vi "Test App Add Process with Used Name Throws Error.vi"(8 "error in (no error)":errorcluster, 11 "Rig Test in":refnum<class "Application Dev Test.lvclass">) -> (0 "error out":errorcluster, 3 "Rig Test out":refnum<class "Application Dev Test.lvclass">)   [LabVIEW 2020, in "Application Dev Test.lvclass"]
uses:
  Application Dev Test.lvclass
  C:/Program Files (x86)/National Instruments/LabVIEW 2020/vi.lib/Astemes/LUnit/Test Case.lvclass
  source/Framework/Process/Process.lvclass
  source/Framework Test Suite/Mock Error Handler/Mock Error Handler.lvclass
  C:/Git/triarc-framework/source/Framework/Error Handler Interface/Error Handler Interface.lvclass
  source/Framework/Process/Process.lvclass/Process.ctl
  source/Framework/Application/Application.lvclass/Application.ctl
  <vilib>/Astemes/LUnit/Test Case.lvclass/Test Case.ctl
  <vilib>/Astemes/LUnit/LUnit Assertion Result.lvclass/LUnit Assertion Result.ctl
  <vilib>/Astemes/LUnit/LUnit Test Case Result.lvclass/LUnit Test Case Result.ctl
  <vilib>/Astemes/LUnit/LUnit Method Result.lvclass/LUnit Method Result.ctl
  b0215dd9-40b6-4c3d-8097-4c1eb93856a7.vi
  source/Framework/Process/Protected/Messaging/Enqueue Message.vi
  source/Framework/Process/Public/Lifecycle/Get Lifecycle State.vi
  source/Framework/Process/Protected/Messaging/Request Message.vi
  source/Framework/Application/Private/Add Process to Map.vi
  source/Framework/Application/Private/Start Idle Processes if Running.vi
  source/Framework/Application/Private/Throw Error If Process Already in App.vi
  source/Framework/Process/Protected/SubVIs/Set Context.vi
  <vilib>/Astemes/LUnit/Palette/Fail.vi
  <vilib>/Astemes/LUnit/Palette/Pass.vi
  <vilib>/Astemes/LUnit/Set Assertion Type.vi
  <vilib>/Astemes/LUnit/Compare Variants.vi
  <vilib>/Astemes/LUnit/Describe Comparison.vi
  source/Framework/Process/Private/SubVIs/Wait for finish.vi
  source/Framework/Process/Private/SubVIs/Set Lifecycle State.vi
  source/Framework/Process/Private/SubVIs/Handle Debug Data.vi
  <vilib>/Utility/error.llb/Clear Errors.vi
  source/Framework/Process/Private/SubVIs/Enqueue Request Message.vi
  source/Framework/Application/Public/Get Process.vi
  source/Framework/Process/Public/Lifecycle/Leave Process Loop.vi
  <vilib>/Astemes/LUnit/Add test result.vi
  <vilib>/Astemes/LUnit/LUnit Write Passed.vi
  <vilib>/Astemes/LUnit/LUnit Write Message.vi
  <vilib>/Astemes/LUnit/LUnit Write Description.vi
  <vilib>/Astemes/LUnit/LUnit Write Assertion Type.vi
  <vilib>/Astemes/LUnit/Variant to string.vi
  source/Framework/Logging/Log Debug.vi
  <vilib>/AdvancedString/1D String Array to Delimited String.vi
  <vilib>/Utility/High Resolution Relative Seconds.vi
  source/Framework/Application/Private/Retrieve Process from App.vi
  source/Framework/Application/Private/Parse Process Name.vi
  source/Framework/Application/Private/Get Process from Map.vi
  <vilib>/Astemes/LUnit/LUnit Record Assertion Result.vi
  <vilib>/AdvancedString/Delimited String to 1D String Array.vi
  <vilib>/Astemes/LUnit/LUnit Aggregate Assertion Results.vi
  <vilib>/Astemes/LUnit/Assertion Result/LUnit Read Status.vi
  <vilib>/Astemes/LUnit/LUnit Read Message.vi
  <vilib>/Astemes/LUnit/LUnit Read Description.vi
  <vilib>/Astemes/LUnit/Method Result/LUnit Merge Status.vi
  <vilib>/Astemes/LUnit/LUnit Concatenate result strings.vi
  source/Framework/Application/Application.lvclass
  C:/Git/triarc-framework/source/Framework/Process/Process.lvclass
  <vilib>/Utility/error.llb/Error Cluster From Error Code.vi
  source/Framework/Process/Public/Read Name.vi
  source/Framework/Process/Private/SubVIs/Wait for Response Message.vi
  <vilib>/Utility/Data Type/Get Type Information.vi
  <vilib>/Utility/LVClass/Get LV Class Name.vi
  <vilib>/Astemes/LUnit/LUnit Assertion Result.lvclass
  <vilib>/Astemes/LUnit/Test Case.lvclass
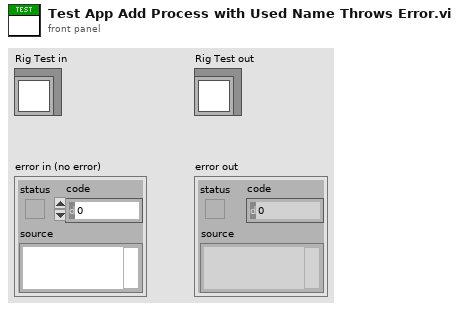
[diagram p1: front panel]
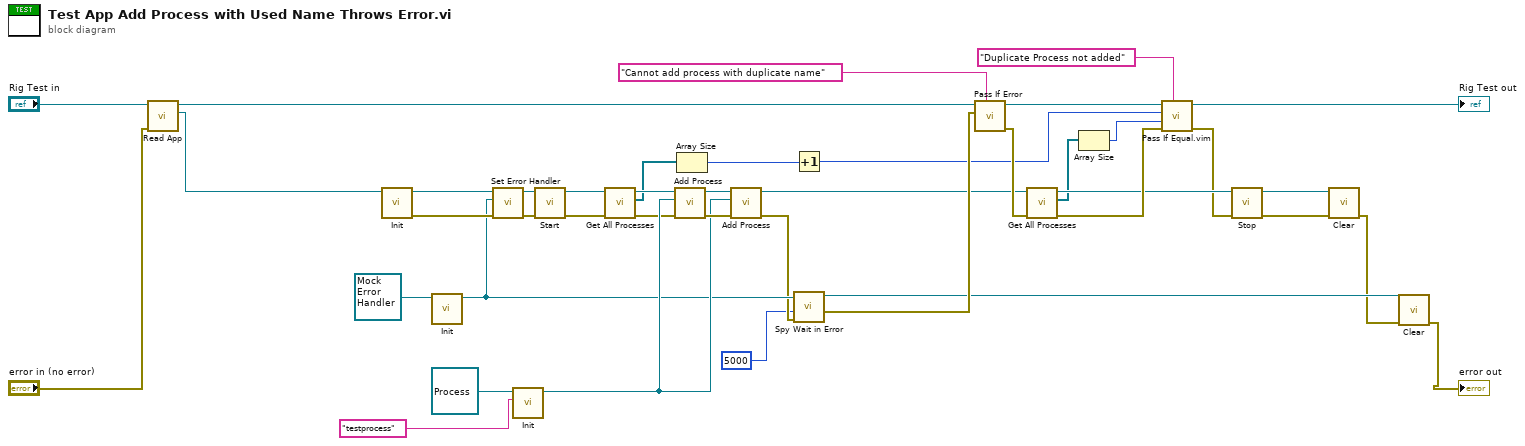
[diagram p0: block diagram]
diagram:
  n1 = call "Read App.vi"("error in (no error)"="error in (no error)", "Application Test In"="Rig Test in") -> ("App out"=w40:refnum<class "Application.lvclass">, "Application Test Out"=w30:refnum<class "Application Dev Test.lvclass">)  [unwired: 7 in, 1 out]
  n2 = call-dynamic "Init.vi"("Process In"=w40) -> ("error out"=w31:errorcluster, "Process Out"=w25:refnum<class "Application.lvclass">)  [unwired: 9 in]
  n3 = call-dynamic "Init.vi"("Mock Error Handler In"=refnum<class "Mock Error Handler.lvclass"> refnum ("Mock Error Handler.lvclass")) -> ("Mock Error Handler Out"=w22:refnum<class "Mock Error Handler.lvclass">)  [unwired: 9 in, 1 out]
  n4 = call "Set Error Handler.vi"("error in (no error)"=w31, "Error Handler"=w22, "Process In"=w25) -> ("error out"=w26:errorcluster, "Process Out"=w24:refnum<class "Application.lvclass">)  [unwired: 7 in]
  n5 = call-dynamic "Init.vi"("Name"="testprocess", "Process In"=refnum<class "Process.lvclass"> refnum ("Process.lvclass")) -> ("Process Out"=w27:refnum<class "Process.lvclass">)  [unwired: 8 in, 1 out]
  n6 = call "Start.vi"("error in (no error)"=w26, "Process In"=w24) -> ("error out"=w32:errorcluster, "Process Out"=w5:refnum<class "Application.lvclass">)  [unwired: 7 in, 1 out]
  n7 = call "Get All Processes.vi"("error in (no error)"=w32, "Application In"=w5) -> ("error out"=w6:errorcluster, "App Processes"=w3:refnum<class "Process.lvclass">[], "Application Out"=w4:refnum<class "Application.lvclass">)  [unwired: 7 in]
  n8 = call "Add Process.vi"("error in (no error)"=w6, "Process"=w27, "Application In"=w4) -> ("error out"=w35:errorcluster, "Application Out"=w38:refnum<class "Application.lvclass">)  [unwired: 7 in]
  n9 = Array Size(array=w3) -> (size(s)=w2:i32)
  n10 = call "Add Process.vi"("error in (no error)"=w35, "Process"=w27, "Application In"=w38) -> ("error out"=w21:errorcluster, "Application Out"=w15:refnum<class "Application.lvclass">)  [unwired: 7 in]
  n11 = Increment(x=w2) -> (x+1=w1:i32)
  n12 = call "Spy Wait in Error.vi"("error in (no error)"=w21, "timeout in ms (-1)"=5000, "Mock Error Handler In"=w22) -> ("Errors"=w20:errorcluster, "Mock Error Handler Out"=w19:refnum<class "Mock Error Handler.lvclass">)  [unwired: 4 in, 3 out]
  n13 = call <vilib>:"Pass If Error.vi"("Description"="Cannot add process with duplicate name", "Assert error"=w20, "LUnit Test Case In"=w30) -> ("error out"=w34:errorcluster, "LUnit Test Case Out"=w12:refnum<class "Application Dev Test.lvclass">)  [unwired: 7 in]
  n14 = call "Get All Processes.vi"("error in (no error)"=w34, "Application In"=w15) -> ("error out"=w16:errorcluster, "App Processes"=w10:refnum<class "Process.lvclass">[], "Application Out"=w14:refnum<class "Application.lvclass">)  [unwired: 7 in]
  n15 = Array Size(array=w10) -> (size(s)=w9:i32)
  n16 = call "Pass If Equal.vim"("Description"="Duplicate Process not added", "error in (no error)"=w16, "Actual"=w9, "Expected"=w1, "LUnit Test Case In"=w12) -> ("error out"=w13:errorcluster, "LUnit Test Case Out"=→"Rig Test out":refnum<class "Application Dev Test.lvclass">)  [unwired: 5 in]
  n17 = call "Stop.vi"("error in (no error)"=w13, "Process In"=w14) -> ("error out"=w29:errorcluster, "Process Out"=w28:refnum<class "Application.lvclass">)  [unwired: 7 in, 1 out]
  n18 = call-dynamic "Clear.vi"("error in (no error)"=w29, "Application In"=w28) -> ("error out"=w18:errorcluster)  [unwired: 9 in]
  n19 = call-dynamic "Clear.vi"("error in (no error)"=w18, "Mock Process In"=w19) -> ("error out"=→"error out":errorcluster)  [unwired: 9 in]
